vi "DDS_Clock.vi"() -> ()   [LabVIEW 2016] (continued)
 [Hz] CH0"=300199999.99999994}, {"total time[ms]"=89.94999999999703, "f1 [Hz] CH0"=300199999.99999994}, {"total time[ms]"=89.99999999999703, "f1 [Hz] CH0"=300000000.0}, {"total time[ms]"=89.99999999999703, "f1 [Hz] CH0"=300000000.0}, {"total time[ms]"=90.04999999999703, "f1 [Hz] CH0"=300200000.00000006}, {"total time[ms]"=90.04999999999703, "f1 [Hz] CH0"=300200000.00000006}, {"total time[ms]"=90.09999999999702, "f1 [Hz] CH0"=300400000.00000006}, {"total time[ms]"=90.09999999999702, "f1 [Hz] CH0"=300400000.00000006}, {"total time[ms]"=90.14999999999702, "f1 [Hz] CH0"=300600000.0}, {"total time[ms]"=90.14999999999702, "f1 [Hz] CH0"=300600000.0}, {"total time[ms]"=90.19999999999702, "f1 [Hz] CH0"=300800000.00000006}, {"total time[ms]"=90.19999999999702, "f1 [Hz] CH0"=300800000.00000006}, {"total time[ms]"=90.24999999999702, "f1 [Hz] CH0"=301000000.0}, {"total time[ms]"=90.24999999999702, "f1 [Hz] CH0"=301000000.0}, {"total time[ms]"=90.29999999999701, "f1 [Hz] CH0"=301200000.00000006}, {"total time[ms]"=90.29999999999701, "f1 [Hz] CH0"=301200000.00000006}, {"total time[ms]"=90.34999999999701, "f1 [Hz] CH0"=301400000.00000006}, {"total time[ms]"=90.34999999999701, "f1 [Hz] CH0"=301400000.00000006}, {"total time[ms]"=90.39999999999701, "f1 [Hz] CH0"=301600000.00000006}, {"total time[ms]"=90.39999999999701, "f1 [Hz] CH0"=301600000.00000006}, {"total time[ms]"=90.449999999997, "f1 [Hz] CH0"=301800000.0}, {"total time[ms]"=90.449999999997, "f1 [Hz] CH0"=301800000.0}, {"total time[ms]"=90.499999999997, "f1 [Hz] CH0"=302000000.0}, {"total time[ms]"=90.499999999997, "f1 [Hz] CH0"=302000000.0}, {"total time[ms]"=90.549999999997, "f1 [Hz] CH0"=302200000.00000006}, {"total time[ms]"=90.549999999997, "f1 [Hz] CH0"=302200000.00000006}, {"total time[ms]"=90.599999999997, "f1 [Hz] CH0"=302400000.0}, {"total time[ms]"=90.599999999997, "f1 [Hz] CH0"=302400000.0}, {"total time[ms]"=90.649999999997, "f1 [Hz] CH0"=302600000.00000006}, {"total time[ms]"=90.649999999997, "f1 [Hz] CH0"=302600000.00000006}, {"total time[ms]"=90.69999999999699, "f1 [Hz] CH0"=302800000.0}, {"total time[ms]"=90.69999999999699, "f1 [Hz] CH0"=302800000.0}, {"total time[ms]"=90.74999999999699, "f1 [Hz] CH0"=303000000.00000006}, {"total time[ms]"=90.74999999999699, "f1 [Hz] CH0"=303000000.00000006}, {"total time[ms]"=90.79999999999698, "f1 [Hz] CH0"=303200000.00000006}, {"total time[ms]"=90.79999999999698, "f1 [Hz] CH0"=303200000.00000006}, {"total time[ms]"=90.84999999999698, "f1 [Hz] CH0"=303400000.00000006}, {"total time[ms]"=90.84999999999698, "f1 [Hz] CH0"=303400000.00000006}, {"total time[ms]"=90.89999999999698, "f1 [Hz] CH0"=303600000.00000006}, {"total time[ms]"=90.89999999999698, "f1 [Hz] CH0"=303600000.00000006}, {"total time[ms]"=90.94999999999698, "f1 [Hz] CH0"=303800000.0}, {"total time[ms]"=90.94999999999698, "f1 [Hz] CH0"=303800000.0}, {"total time[ms]"=90.99999999999697, "f1 [Hz] CH0"=304000000.0}, {"total time[ms]"=90.99999999999697, "f1 [Hz] CH0"=304000000.0}, {"total time[ms]"=91.04999999999697, "f1 [Hz] CH0"=304200000.00000006}, {"total time[ms]"=91.04999999999697, "f1 [Hz] CH0"=304200000.00000006}, {"total time[ms]"=91.09999999999697, "f1 [Hz] CH0"=304400000.00000006}, {"total time[ms]"=91.09999999999697, "f1 [Hz] CH0"=304400000.00000006}, {"total time[ms]"=91.14999999999696, "f1 [Hz] CH0"=304600000.0}, {"total time[ms]"=91.14999999999696, "f1 [Hz] CH0"=304600000.0}, {"total time[ms]"=91.19999999999696, "f1 [Hz] CH0"=304800000.00000006}, {"total time[ms]"=91.19999999999696, "f1 [Hz] CH0"=304800000.00000006}, {"total time[ms]"=91.24999999999696, "f1 [Hz] CH0"=305000000.0}, {"total time[ms]"=91.24999999999696, "f1 [Hz] CH0"=305000000.0}, {"total time[ms]"=91.29999999999696, "f1 [Hz] CH0"=305200000.00000006}, {"total time[ms]"=91.29999999999696, "f1 [Hz] CH0"=305200000.00000006}, {"total time[ms]"=91.34999999999695, "f1 [Hz] CH0"=305400000.00000006}, {"total time[ms]"=91.34999999999695, "f1 [Hz] CH0"=305400000.00000006}, {"total time[ms]"=91.39999999999695, "f1 [Hz] CH0"=305600000.0}, {"total time[ms]"=91.39999999999695, "f1 [Hz] CH0"=305600000.0}, {"total time[ms]"=91.44999999999695, "f1 [Hz] CH0"=305800000.00000006}, {"total time[ms]"=91.44999999999695, "f1 [Hz] CH0"=305800000.00000006}, {"total time[ms]"=91.49999999999694, "f1 [Hz] CH0"=306000000.0}, {"total time[ms]"=91.49999999999694, "f1 [Hz] CH0"=306000000.0}, {"total time[ms]"=91.54999999999694, "f1 [Hz] CH0"=306200000.00000006}, {"total time[ms]"=91.54999999999694, "f1 [Hz] CH0"=306200000.00000006}, {"total time[ms]"=91.59999999999694, "f1 [Hz] CH0"=306400000.00000006}, {"total time[ms]"=91.59999999999694, "f1 [Hz] CH0"=306400000.00000006}, {"total time[ms]"=91.64999999999694, "f1 [Hz] CH0"=306600000.00000006}, {"total time[ms]"=91.64999999999694, "f1 [Hz] CH0"=306600000.00000006}, {"total time[ms]"=91.69999999999693, "f1 [Hz] CH0"=306800000.0}, {"total time[ms]"=91.69999999999693, "f1 [Hz] CH0"=306800000.0}, {"total time[ms]"=91.74999999999693, "f1 [Hz] CH0"=307000000.0}, {"total time[ms]"=91.74999999999693, "f1 [Hz] CH0"=307000000.0}, {"total time[ms]"=91.79999999999693, "f1 [Hz] CH0"=307200000.00000006}, {"total time[ms]"=91.79999999999693, "f1 [Hz] CH0"=307200000.00000006}, {"total time[ms]"=91.84999999999692, "f1 [Hz] CH0"=307400000.0}, {"total time[ms]"=91.84999999999692, "f1 [Hz] CH0"=307400000.0}, {"total time[ms]"=91.89999999999692, "f1 [Hz] CH0"=307600000.00000006}, {"total time[ms]"=91.89999999999692, "f1 [Hz] CH0"=307600000.00000006}, {"total time[ms]"=91.94999999999692, "f1 [Hz] CH0"=307800000.0}, {"total time[ms]"=91.94999999999692, "f1 [Hz] CH0"=307800000.0}, {"total time[ms]"=91.99999999999692, "f1 [Hz] CH0"=308000000.00000006}, {"total time[ms]"=91.99999999999692, "f1 [Hz] CH0"=308000000.00000006}, {"total time[ms]"=92.04999999999691, "f1 [Hz] CH0"=308200000.00000006}, {"total time[ms]"=92.04999999999691, "f1 [Hz] CH0"=308200000.00000006}, {"total time[ms]"=92.09999999999691, "f1 [Hz] CH0"=308400000.00000006}, {"total time[ms]"=92.09999999999691, "f1 [Hz] CH0"=308400000.00000006}, {"total time[ms]"=92.14999999999691, "f1 [Hz] CH0"=308600000.00000006}, {"total time[ms]"=92.14999999999691, "f1 [Hz] CH0"=308600000.00000006}, {"total time[ms]"=92.1999999999969, "f1 [Hz] CH0"=308800000.0}, {"total time[ms]"=92.1999999999969, "f1 [Hz] CH0"=308800000.0}, {"total time[ms]"=92.2499999999969, "f1 [Hz] CH0"=309000000.0}, {"total time[ms]"=92.2499999999969, "f1 [Hz] CH0"=309000000.0}, {"total time[ms]"=92.2999999999969, "f1 [Hz] CH0"=309200000.00000006}, {"total time[ms]"=92.2999999999969, "f1 [Hz] CH0"=309200000.00000006}, {"total time[ms]"=92.3499999999969, "f1 [Hz] CH0"=309400000.00000006}, {"total time[ms]"=92.3499999999969, "f1 [Hz] CH0"=309400000.00000006}, {"total time[ms]"=92.3999999999969, "f1 [Hz] CH0"=309600000.0}, {"total time[ms]"=92.3999999999969, "f1 [Hz] CH0"=309600000.0}, {"total time[ms]"=92.44999999999689, "f1 [Hz] CH0"=309800000.00000006}, {"total time[ms]"=92.44999999999689, "f1 [Hz] CH0"=309800000.00000006}, {"total time[ms]"=92.49999999999689, "f1 [Hz] CH0"=310000000.0}, {"total time[ms]"=92.49999999999689, "f1 [Hz] CH0"=310000000.0}, {"total time[ms]"=92.54999999999688, "f1 [Hz] CH0"=310200000.00000006}, {"total time[ms]"=92.54999999999688, "f1 [Hz] CH0"=310200000.00000006}, {"total time[ms]"=92.59999999999688, "f1 [Hz] CH0"=310400000.00000006}, {"total time[ms]"=92.59999999999688, "f1 [Hz] CH0"=310400000.00000006}, {"total time[ms]"=92.64999999999688, "f1 [Hz] CH0"=310600000.0}, {"total time[ms]"=92.64999999999688, "f1 [Hz] CH0"=310600000.0}, {"total time[ms]"=92.69999999999688, "f1 [Hz] CH0"=310800000.00000006}, {"total time[ms]"=92.69999999999688, "f1 [Hz] CH0"=310800000.00000006}, {"total time[ms]"=92.74999999999687, "f1 [Hz] CH0"=311000000.0}, {"total time[ms]"=92.74999999999687, "f1 [Hz] CH0"=311000000.0}, {"total time[ms]"=92.79999999999687, "f1 [Hz] CH0"=311200000.00000006}, {"total time[ms]"=92.79999999999687, "f1 [Hz] CH0"=311200000.00000006}, {"total time[ms]"=92.84999999999687, "f1 [Hz] CH0"=311400000.00000006}, {"total time[ms]"=92.84999999999687, "f1 [Hz] CH0"=311400000.00000006}, {"total time[ms]"=92.89999999999687, "f1 [Hz] CH0"=311600000.00000006}, {"total time[ms]"=92.89999999999687, "f1 [Hz] CH0"=311600000.00000006}, {"total time[ms]"=92.94999999999686, "f1 [Hz] CH0"=311800000.0}, {"total time[ms]"=92.94999999999686, "f1 [Hz] CH0"=311800000.0}, {"total time[ms]"=92.99999999999686, "f1 [Hz] CH0"=312000000.0}, {"total time[ms]"=92.99999999999686, "f1 [Hz] CH0"=312000000.0}, {"total time[ms]"=93.04999999999686, "f1 [Hz] CH0"=312200000.00000006}, {"total time[ms]"=93.04999999999686, "f1 [Hz] CH0"=312200000.00000006}, {"total time[ms]"=93.09999999999685, "f1 [Hz] CH0"=312400000.0}, {"total time[ms]"=93.09999999999685, "f1 [Hz] CH0"=312400000.0}, {"total time[ms]"=93.14999999999685, "f1 [Hz] CH0"=312600000.00000006}, {"total time[ms]"=93.14999999999685, "f1 [Hz] CH0"=312600000.00000006}, {"total time[ms]"=93.19999999999685, "f1 [Hz] CH0"=312800000.0}, {"total time[ms]"=93.19999999999685, "f1 [Hz] CH0"=312800000.0}, {"total time[ms]"=93.24999999999685, "f1 [Hz] CH0"=313000000.00000006}, {"total time[ms]"=93.24999999999685, "f1 [Hz] CH0"=313000000.00000006}, {"total time[ms]"=93.29999999999684, "f1 [Hz] CH0"=313200000.00000006}, {"total time[ms]"=93.29999999999684, "f1 [Hz] CH0"=313200000.00000006}, {"total time[ms]"=93.34999999999684, "f1 [Hz] CH0"=313400000.00000006}, {"total time[ms]"=93.34999999999684, "f1 [Hz] CH0"=313400000.00000006}, {"total time[ms]"=93.39999999999684, "f1 [Hz] CH0"=313600000.00000006}, {"total time[ms]"=93.39999999999684, "f1 [Hz] CH0"=313600000.00000006}, {"total time[ms]"=93.44999999999683, "f1 [Hz] CH0"=313800000.0}, {"total time[ms]"=93.44999999999683, "f1 [Hz] CH0"=313800000.0}, {"total time[ms]"=93.49999999999683, "f1 [Hz] CH0"=314000000.0}, {"total time[ms]"=93.49999999999683, "f1 [Hz] CH0"=314000000.0}, {"total time[ms]"=93.54999999999683, "f1 [Hz] CH0"=314200000.00000006}, {"total time[ms]"=93.54999999999683, "f1 [Hz] CH0"=314200000.00000006}, {"total time[ms]"=93.59999999999683, "f1 [Hz] CH0"=314400000.00000006}, {"total time[ms]"=93.59999999999683, "f1 [Hz] CH0"=314400000.00000006}, {"total time[ms]"=93.64999999999682, "f1 [Hz] CH0"=314600000.0}, {"total time[ms]"=93.64999999999682, "f1 [Hz] CH0"=314600000.0}, {"total time[ms]"=93.69999999999682, "f1 [Hz] CH0"=314800000.00000006}, {"total time[ms]"=93.69999999999682, "f1 [Hz] CH0"=314800000.00000006}, {"total time[ms]"=93.74999999999682, "f1 [Hz] CH0"=315000000.0}, {"total time[ms]"=93.74999999999682, "f1 [Hz] CH0"=315000000.0}, {"total time[ms]"=93.79999999999681, "f1 [Hz] CH0"=315200000.00000006}, {"total time[ms]"=93.79999999999681, "f1 [Hz] CH0"=315200000.00000006}, {"total time[ms]"=93.84999999999681, "f1 [Hz] CH0"=315400000.00000006}, {"total time[ms]"=93.84999999999681, "f1 [Hz] CH0"=315400000.00000006}, {"total time[ms]"=93.89999999999681, "f1 [Hz] CH0"=315600000.0}, {"total time[ms]"=93.89999999999681, "f1 [Hz] CH0"=315600000.0}, {"total time[ms]"=93.9499999999968, "f1 [Hz] CH0"=315800000.00000006}, {"total time[ms]"=93.9499999999968, "f1 [Hz] CH0"=315800000.00000006}, {"total time[ms]"=93.9999999999968, "f1 [Hz] CH0"=316000000.0}, {"total time[ms]"=93.9999999999968, "f1 [Hz] CH0"=316000000.0}, {"total time[ms]"=94.0499999999968, "f1 [Hz] CH0"=316200000.00000006}, {"total time[ms]"=94.0499999999968, "f1 [Hz] CH0"=316200000.00000006}, {"total time[ms]"=94.0999999999968, "f1 [Hz] CH0"=316400000.00000006}, {"total time[ms]"=94.0999999999968, "f1 [Hz] CH0"=316400000.00000006}, {"total time[ms]"=94.1499999999968, "f1 [Hz] CH0"=316600000.00000006}, {"total time[ms]"=94.1499999999968, "f1 [Hz] CH0"=316600000.00000006}, {"total time[ms]"=94.19999999999679, "f1 [Hz] CH0"=316800000.0}, {"total time[ms]"=94.19999999999679, "f1 [Hz] CH0"=316800000.0}, {"total time[ms]"=94.24999999999679, "f1 [Hz] CH0"=317000000.0}, {"total time[ms]"=94.24999999999679, "f1 [Hz] CH0"=317000000.0}, {"total time[ms]"=94.29999999999679, "f1 [Hz] CH0"=317200000.00000006}, {"total time[ms]"=94.29999999999679, "f1 [Hz] CH0"=317200000.00000006}, {"total time[ms]"=94.34999999999678, "f1 [Hz] CH0"=317400000.0}, {"total time[ms]"=94.34999999999678, "f1 [Hz] CH0"=317400000.0}, {"total time[ms]"=94.39999999999678, "f1 [Hz] CH0"=317600000.00000006}, {"total time[ms]"=94.39999999999678, "f1 [Hz] CH0"=317600000.00000006}, {"total time[ms]"=94.44999999999678, "f1 [Hz] CH0"=317800000.0}, {"total time[ms]"=94.44999999999678, "f1 [Hz] CH0"=317800000.0}, {"total time[ms]"=94.49999999999677, "f1 [Hz] CH0"=318000000.00000006}, {"total time[ms]"=94.49999999999677, "f1 [Hz] CH0"=318000000.00000006}, {"total time[ms]"=94.54999999999677, "f1 [Hz] CH0"=318200000.00000006}, {"total time[ms]"=94.54999999999677, "f1 [Hz] CH0"=318200000.00000006}, {"total time[ms]"=94.59999999999677, "f1 [Hz] CH0"=318400000.00000006}, {"total time[ms]"=94.59999999999677, "f1 [Hz] CH0"=318400000.00000006}, {"total time[ms]"=94.64999999999677, "f1 [Hz] CH0"=318600000.00000006}, {"total time[ms]"=94.64999999999677, "f1 [Hz] CH0"=318600000.00000006}, {"total time[ms]"=94.69999999999676, "f1 [Hz] CH0"=318800000.0}, {"total time[ms]"=94.69999999999676, "f1 [Hz] CH0"=318800000.0}, {"total time[ms]"=94.74999999999676, "f1 [Hz] CH0"=319000000.0}, {"total time[ms]"=94.74999999999676, "f1 [Hz] CH0"=319000000.0}, {"total time[ms]"=94.79999999999676, "f1 [Hz] CH0"=319200000.0000001}, {"total time[ms]"=94.79999999999676, "f1 [Hz] CH0"=319200000.0000001}, {"total time[ms]"=94.84999999999675, "f1 [Hz] CH0"=319400000.00000006}, {"total time[ms]"=94.84999999999675, "f1 [Hz] CH0"=319400000.00000006}, {"total time[ms]"=94.89999999999675, "f1 [Hz] CH0"=319600000.0}, {"total time[ms]"=94.89999999999675, "f1 [Hz] CH0"=319600000.0}, {"total time[ms]"=94.94999999999675, "f1 [Hz] CH0"=319800000.00000006}, {"total time[ms]"=94.94999999999675, "f1 [Hz] CH0"=319800000.00000006}, {"total time[ms]"=94.99999999999675, "f1 [Hz] CH0"=320000000.0}, {"total time[ms]"=94.99999999999675, "f1 [Hz] CH0"=320000000.0}, {"total time[ms]"=95.04999999999674, "f1 [Hz] CH0"=319800000.0}, {"total time[ms]"=95.04999999999674, "f1 [Hz] CH0"=319800000.0}, {"total time[ms]"=95.09999999999674, "f1 [Hz] CH0"=319599999.99999994}, {"total time[ms]"=95.09999999999674, "f1 [Hz] CH0"=319599999.99999994}, {"total time[ms]"=95.14999999999674, "f1 [Hz] CH0"=319400000.0}, {"total time[ms]"=95.14999999999674, "f1 [Hz] CH0"=319400000.0}, {"total time[ms]"=95.19999999999673, "f1 [Hz] CH0"=319199999.99999994}, {"total time[ms]"=95.19999999999673, "f1 [Hz] CH0"=319199999.99999994}, {"total time[ms]"=95.24999999999673, "f1 [Hz] CH0"=319000000.0}, {"total time[ms]"=95.24999999999673, "f1 [Hz] CH0"=319000000.0}, {"total time[ms]"=95.29999999999673, "f1 [Hz] CH0"=318799999.99999994}, {"total time[ms]"=95.29999999999673, "f1 [Hz] CH0"=318799999.99999994}, {"total time[ms]"=95.34999999999673, "f1 [Hz] CH0"=318599999.99999994}, {"total time[ms]"=95.34999999999673, "f1 [Hz] CH0"=318599999.99999994}, {"total time[ms]"=95.39999999999672, "f1 [Hz] CH0"=318399999.99999994}, {"total time[ms]"=95.39999999999672, "f1 [Hz] CH0"=318399999.99999994}, {"total time[ms]"=95.44999999999672, "f1 [Hz] CH0"=318200000.0}, {"total time[ms]"=95.44999999999672, "f1 [Hz] CH0"=318200000.0}, {"total time[ms]"=95.49999999999672, "f1 [Hz] CH0"=318000000.0}, {"total time[ms]"=95.49999999999672, "f1 [Hz] CH0"=318000000.0}, {"total time[ms]"=95.54999999999671, "f1 [Hz] CH0"=317799999.99999994}, {"total time[ms]"=95.54999999999671, "f1 [Hz] CH0"=317799999.99999994}, {"total time[ms]"=95.59999999999671, "f1 [Hz] CH0"=317600000.0}, {"total time[ms]"=95.59999999999671, "f1 [Hz] CH0"=317600000.0}, {"total time[ms]"=95.64999999999671, "f1 [Hz] CH0"=317399999.99999994}, {"total time[ms]"=95.64999999999671, "f1 [Hz] CH0"=317399999.99999994}, {"total time[ms]"=95.6999999999967, "f1 [Hz] CH0"=317200000.0}, {"total time[ms]"=95.6999999999967, "f1 [Hz] CH0"=317200000.0}, {"total time[ms]"=95.7499999999967, "f1 [Hz] CH0"=316999999.99999994}, {"total time[ms]"=95.7499999999967, "f1 [Hz] CH0"=316999999.99999994}, {"total time[ms]"=95.7999999999967, "f1 [Hz] CH0"=316799999.99999994}, {"total time[ms]"=95.7999999999967, "f1 [Hz] CH0"=316799999.99999994}, {"total time[ms]"=95.8499999999967, "f1 [Hz] CH0"=316599999.99999994}, {"total time[ms]"=95.8499999999967, "f1 [Hz] CH0"=316599999.99999994}, {"total time[ms]"=95.8999999999967, "f1 [Hz] CH0"=316399999.99999994}, {"total time[ms]"=95.8999999999967, "f1 [Hz] CH0"=316399999.99999994}, {"total time[ms]"=95.94999999999669, "f1 [Hz] CH0"=316200000.0}, {"total time[ms]"=95.94999999999669, "f1 [Hz] CH0"=316200000.0}, {"total time[ms]"=95.99999999999669, "f1 [Hz] CH0"=315999999.99999994}, {"total time[ms]"=95.99999999999669, "f1 [Hz] CH0"=315999999.99999994}, {"total time[ms]"=96.04999999999669, "f1 [Hz] CH0"=315799999.99999994}, {"total time[ms]"=96.04999999999669, "f1 [Hz] CH0"=315799999.99999994}, {"total time[ms]"=96.09999999999668, "f1 [Hz] CH0"=315599999.99999994}, {"total time[ms]"=96.09999999999668, "f1 [Hz] CH0"=315599999.99999994}, {"total time[ms]"=96.14999999999668, "f1 [Hz] CH0"=315399999.99999994}, {"total time[ms]"=96.14999999999668, "f1 [Hz] CH0"=315399999.99999994}, {"total time[ms]"=96.19999999999668, "f1 [Hz] CH0"=315199999.99999994}, {"total time[ms]"=96.19999999999668, "f1 [Hz] CH0"=315199999.99999994}, {"total time[ms]"=96.24999999999667, "f1 [Hz] CH0"=315000000.0}, {"total time[ms]"=96.24999999999667, "f1 [Hz] CH0"=315000000.0}, {"total time[ms]"=96.29999999999667, "f1 [Hz] CH0"=314799999.9999999}, {"total time[ms]"=96.29999999999667, "f1 [Hz] CH0"=314799999.9999999}, {"total time[ms]"=96.34999999999667, "f1 [Hz] CH0"=314599999.99999994}, {"total time[ms]"=96.34999999999667, "f1 [Hz] CH0"=314599999.99999994}, {"total time[ms]"=96.39999999999667, "f1 [Hz] CH0"=314400000.0}, {"total time[ms]"=96.39999999999667, "f1 [Hz] CH0"=314400000.0}, {"total time[ms]"=96.44999999999666, "f1 [Hz] CH0"=314199999.99999994}, {"total time[ms]"=96.44999999999666, "f1 [Hz] CH0"=314199999.99999994}, {"total time[ms]"=96.49999999999666, "f1 [Hz] CH0"=314000000.0}, {"total time[ms]"=96.49999999999666, "f1 [Hz] CH0"=314000000.0}, {"total time[ms]"=96.54999999999666, "f1 [Hz] CH0"=313799999.99999994}, {"total time[ms]"=96.54999999999666, "f1 [Hz] CH0"=313799999.99999994}, {"total time[ms]"=96.59999999999665, "f1 [Hz] CH0"=313599999.99999994}, {"total time[ms]"=96.59999999999665, "f1 [Hz] CH0"=313599999.99999994}, {"total time[ms]"=96.64999999999665, "f1 [Hz] CH0"=313399999.99999994}, {"total time[ms]"=96.64999999999665, "f1 [Hz] CH0"=313399999.99999994}, {"total time[ms]"=96.69999999999665, "f1 [Hz] CH0"=313199999.99999994}, {"total time[ms]"=96.69999999999665, "f1 [Hz] CH0"=313199999.99999994}, {"total time[ms]"=96.74999999999665, "f1 [Hz] CH0"=313000000.0}, {"total time[ms]"=96.74999999999665, "f1 [Hz] CH0"=313000000.0}, {"total time[ms]"=96.79999999999664, "f1 [Hz] CH0"=312799999.99999994}, {"total time[ms]"=96.79999999999664, "f1 [Hz] CH0"=312799999.99999994}, {"total time[ms]"=96.84999999999664, "f1 [Hz] CH0"=312599999.9999999}, {"total time[ms]"=96.84999999999664, "f1 [Hz] CH0"=312599999.9999999}, {"total time[ms]"=96.89999999999664, "f1 [Hz] CH0"=312399999.99999994}, {"total time[ms]"=96.89999999999664, "f1 [Hz] CH0"=312399999.99999994}, {"total time[ms]"=96.94999999999663, "f1 [Hz] CH0"=312200000.0}, {"total time[ms]"=96.94999999999663, "f1 [Hz] CH0"=312200000.0}, {"total time[ms]"=96.99999999999663, "f1 [Hz] CH0"=311999999.99999994}, {"total time[ms]"=96.99999999999663, "f1 [Hz] CH0"=311999999.99999994}, {"total time[ms]"=97.04999999999663, "f1 [Hz] CH0"=311799999.99999994}, {"total time[ms]"=97.04999999999663, "f1 [Hz] CH0"=311799999.99999994}, {"total time[ms]"=97.09999999999663, "f1 [Hz] CH0"=311599999.99999994}, {"total time[ms]"=97.09999999999663, "f1 [Hz] CH0"=311599999.99999994}, {"total time[ms]"=97.14999999999662, "f1 [Hz] CH0"=311399999.99999994}, {"total time[ms]"=97.14999999999662, "f1 [Hz] CH0"=311399999.99999994}, {"total time[ms]"=97.19999999999662, "f1 [Hz] CH0"=311200000.0}, {"total time[ms]"=97.19999999999662, "f1 [Hz] CH0"=311200000.0}, {"total time[ms]"=97.24999999999662, "f1 [Hz] CH0"=310999999.99999994}, {"total time[ms]"=97.24999999999662, "f1 [Hz] CH0"=310999999.99999994}, {"total time[ms]"=97.29999999999661, "f1 [Hz] CH0"=310799999.99999994}, {"total time[ms]"=97.29999999999661, "f1 [Hz] CH0"=310799999.99999994}, {"total time[ms]"=97.34999999999661, "f1 [Hz] CH0"=310599999.99999994}, {"total time[ms]"=97.34999999999661, "f1 [Hz] CH0"=310599999.99999994}, {"total time[ms]"=97.39999999999661, "f1 [Hz] CH0"=310399999.99999994}, {"total time[ms]"=97.39999999999661, "f1 [Hz] CH0"=310399999.99999994}, {"total time[ms]"=97.4499999999966, "f1 [Hz] CH0"=310199999.99999994}, {"total time[ms]"=97.4499999999966, "f1 [Hz] CH0"=310199999.99999994}, {"total time[ms]"=97.4999999999966, "f1 [Hz] CH0"=310000000.0}, {"total time[ms]"=97.4999999999966, "f1 [Hz] CH0"=310000000.0}, {"total time[ms]"=97.5499999999966, "f1 [Hz] CH0"=309799999.9999999}, {"total time[ms]"=97.5499999999966, "f1 [Hz] CH0"=309799999.9999999}, {"total time[ms]"=97.5999999999966, "f1 [Hz] CH0"=309599999.99999994}, {"total time[ms]"=97.5999999999966, "f1 [Hz] CH0"=309599999.99999994}, {"total time[ms]"=97.6499999999966, "f1 [Hz] CH0"=309400000.0}, {"total time[ms]"=97.6499999999966, "f1 [Hz] CH0"=309400000.0}, {"total time[ms]"=97.69999999999659, "f1 [Hz] CH0"=309199999.99999994}, {"total time[ms]"=97.69999999999659, "f1 [Hz] CH0"=309199999.99999994}, {"total time[ms]"=97.74999999999659, "f1 [Hz] CH0"=309000000.0}, {"total time[ms]"=97.74999999999659, "f1 [Hz] CH0"=309000000.0}, {"total time[ms]"=97.79999999999659, "f1 [Hz] CH0"=308799999.99999994}, {"total time[ms]"=97.79999999999659, "f1 [Hz] CH0"=308799999.99999994}, {"total time[ms]"=97.84999999999658, "f1 [Hz] CH0"=308599999.99999994}, {"total time[ms]"=97.84999999999658, "f1 [Hz] CH0"=308599999.99999994}, {"total time[ms]"=97.89999999999658, "f1 [Hz] CH0"=308399999.99999994}, {"total time[ms]"=97.89999999999658, "f1 [Hz] CH0"=308399999.99999994}, {"total time[ms]"=97.94999999999658, "f1 [Hz] CH0"=308199999.99999994}, {"total time[ms]"=97.94999999999658, "f1 [Hz] CH0"=308199999.99999994}, {"total time[ms]"=97.99999999999658, "f1 [Hz] CH0"=308000000.0}, {"total time[ms]"=97.99999999999658, "f1 [Hz] CH0"=308000000.0}, {"total time[ms]"=98.04999999999657, "f1 [Hz] CH0"=307799999.99999994}, {"total time[ms]"=98.04999999999657, "f1 [Hz] CH0"=307799999.99999994}, {"total time[ms]"=98.09999999999657, "f1 [Hz] CH0"=307599999.9999999}, {"total time[ms]"=98.09999999999657, "f1 [Hz] CH0"=307599999.9999999}, {"total time[ms]"=98.14999999999657, "f1 [Hz] CH0"=307399999.99999994}, {"total time[ms]"=98.14999999999657, "f1 [Hz] CH0"=307399999.99999994}, {"total time[ms]"=98.19999999999656, "f1 [Hz] CH0"=307200000.0}, {"total time[ms]"=98.19999999999656, "f1 [Hz] CH0"=307200000.0}, {"total time[ms]"=98.24999999999656, "f1 [Hz] CH0"=306999999.99999994}, {"total time[ms]"=98.24999999999656, "f1 [Hz] CH0"=306999999.99999994}, {"total time[ms]"=98.29999999999656, "f1 [Hz] CH0"=306799999.99999994}, {"total time[ms]"=98.29999999999656, "f1 [Hz] CH0"=306799999.99999994}, {"total time[ms]"=98.34999999999656, "f1 [Hz] CH0"=306599999.99999994}, {"total time[ms]"=98.34999999999656, "f1 [Hz] CH0"=306599999.99999994}, {"total time[ms]"=98.39999999999655, "f1 [Hz] CH0"=306399999.99999994}, {"total time[ms]"=98.39999999999655, "f1 [Hz] CH0"=306399999.99999994}, {"total time[ms]"=98.44999999999655, "f1 [Hz] CH0"=306200000.0}, {"total time[ms]"=98.44999999999655, "f1 [Hz] CH0"=306200000.0}, {"total time[ms]"=98.49999999999655, "f1 [Hz] CH0"=305999999.99999994}, {"total time[ms]"=98.49999999999655, "f1 [Hz] CH0"=305999999.99999994}, {"total time[ms]"=98.54999999999654, "f1 [Hz] CH0"=305799999.99999994}, {"total time[ms]"=98.54999999999654, "f1 [Hz] CH0"=305799999.99999994}, {"total time[ms]"=98.59999999999654, "f1 [Hz] CH0"=305599999.99999994}, {"total time[ms]"=98.59999999999654, "f1 [Hz] CH0"=305599999.99999994}, {"total time[ms]"=98.64999999999654, "f1 [Hz] CH0"=305399999.99999994}, {"total time[ms]"=98.64999999999654, "f1 [Hz] CH0"=305399999.99999994}, {"total time[ms]"=98.69999999999654, "f1 [Hz] CH0"=305199999.99999994}, {"total time[ms]"=98.69999999999654, "f1 [Hz] CH0"=305199999.99999994}, {"total time[ms]"=98.74999999999653, "f1 [Hz] CH0"=305000000.0}, {"total time[ms]"=98.74999999999653, "f1 [Hz] CH0"=305000000.0}, {"total time[ms]"=98.79999999999653, "f1 [Hz] CH0"=304799999.9999999}, {"total time[ms]"=98.79999999999653, "f1 [Hz] CH0"=304799999.9999999}, {"total time[ms]"=98.84999999999653, "f1 [Hz] CH0"=304599999.99999994}, {"total time[ms]"=98.84999999999653, "f1 [Hz] CH0"=304599999.99999994}, {"total time[ms]"=98.89999999999652, "f1 [Hz] CH0"=304400000.0}, {"total time[ms]"=98.89999999999652, "f1 [Hz] CH0"=304400000.0}, {"total time[ms]"=98.94999999999652, "f1 [Hz] CH0"=304199999.99999994}, {"total time[ms]"=98.94999999999652, "f1 [Hz] CH0"=304199999.99999994}, {"total time[ms]"=98.99999999999652, "f1 [Hz] CH0"=304000000.0}, {"total time[ms]"=98.99999999999652, "f1 [Hz] CH0"=304000000.0}, {"total time[ms]"=99.04999999999652, "f1 [Hz] CH0"=303799999.99999994}, {"total time[ms]"=99.04999999999652, "f1 [Hz] CH0"=303799999.99999994}, {"total time[ms]"=99.09999999999651, "f1 [Hz] CH0"=303599999.99999994}, {"total time[ms]"=99.09999999999651, "f1 [Hz] CH0"=303599999.99999994}, {"total time[ms]"=99.14999999999651, "f1 [Hz] CH0"=303399999.99999994}, {"total time[ms]"=99.14999999999651, "f1 [Hz] CH0"=303399999.99999994}, {"total time[ms]"=99.1999999999965, "f1 [Hz] CH0"=303199999.99999994}, {"total time[ms]"=99.1999999999965, "f1 [Hz] CH0"=303199999.99999994}, {"total time[ms]"=99.2499999999965, "f1 [Hz] CH0"=303000000.0}, {"total time[ms]"=99.2499999999965, "f1 [Hz] CH0"=303000000.0}, {"total time[ms]"=99.2999999999965, "f1 [Hz] CH0"=302799999.99999994}, {"total time[ms]"=99.2999999999965, "f1 [Hz] CH0"=302799999.99999994}, {"total time[ms]"=99.3499999999965, "f1 [Hz] CH0"=302599999.9999999}, {"total time[ms]"=99.3499999999965, "f1 [Hz] CH0"=302599999.9999999}, {"total time[ms]"=99.3999999999965, "f1 [Hz] CH0"=302399999.99999994}, {"total time[ms]"=99.3999999999965, "f1 [Hz] CH0"=302399999.99999994}, {"total time[ms]"=99.44999999999649, "f1 [Hz] CH0"=302200000.0}, {"total time[ms]"=99.44999999999649, "f1 [Hz] CH0"=302200000.0}, {"total time[ms]"=99.49999999999649, "f1 [Hz] CH0"=301999999.99999994}, {"total time[ms]"=99.49999999999649, "f1 [Hz] CH0"=301999999.99999994}, {"total time[ms]"=99.54999999999649, "f1 [Hz] CH0"=301799999.99999994}, {"total time[ms]"=99.54999999999649, "f1 [Hz] CH0"=301799999.99999994}, {"total time[ms]"=99.59999999999648, "f1 [Hz] CH0"=301599999.99999994}, {"total time[ms]"=99.59999999999648, "f1 [Hz] CH0"=301599999.99999994}, {"total time[ms]"=99.64999999999648, "f1 [Hz] CH0"=301399999.99999994}, {"total time[ms]"=99.64999999999648, "f1 [Hz] CH0"=301399999.99999994}, {"total time[ms]"=99.69999999999648, "f1 [Hz] CH0"=301200000.0}, {"total time[ms]"=99.69999999999648, "f1 [Hz] CH0"=301200000.0}, {"total time[ms]"=99.74999999999648, "f1 [Hz] CH0"=300999999.99999994}, {"total time[ms]"=99.74999999999648, "f1 [Hz] CH0"=300999999.99999994}, {"total time[ms]"=99.79999999999647, "f1 [Hz] CH0"=300799999.99999994}, {"total time[ms]"=99.79999999999647, "f1 [Hz] CH0"=300799999.99999994}, {"total time[ms]"=99.84999999999647, "f1 [Hz] CH0"=300599999.99999994}, {"total time[ms]"=99.84999999999647, "f1 [Hz] CH0"=300599999.99999994}, {"total time[ms]"=99.89999999999647, "f1 [Hz] CH0"=300399999.99999994}, {"total time[ms]"=99.89999999999647, "f1 [Hz] CH0"=300399999.99999994}, {"total time[ms]"=99.94999999999646, "f1 [Hz] CH0"=300199999.99999994}, {"total time[ms]"=99.94999999999646, "f1 [Hz] CH0"=300199999.99999994}, {"total time[ms]"=99.99999999999646, "f1 [Hz] CH0"=300000000.0}, {"total time[ms]"=99.99999999999646, "f1 [Hz] CH0"=300000000.0}, {"total time[ms]"=100.04999999999646, "f1 [Hz] CH0"=300200000.0000001}]}, ...(2 in all)]
  in  "Store data":enum32{"Save settings", "Don't save settings"}(tab)=enum."Don't save settings"
  in  "XML File Path WRITE":path=path "U:/Dokumente/Bachelorarbeit/Labview/FlexDDS-NG/conf/settings_s_curve_up_down.xml"
  in  "Select curve form":enum32{"Triangular", "Sinusodial"}(ring)
  in  "Single Frequency (MHz)":dbl=310.0 format="%#_13g"
  in  "Channel - Constant":T7(ring)
  in  "Ramping Parameters":T8={"Number of steps"=2000, "Total Time (ms)"=100.0, "Start frequency (MHz)"=300.0, "End frequency (MHz)"=320.0, "Cycle Time (ms)"=10.0} {"Cycle Time (ms)" format="%#_13g"}
  # "Channel - Ramp"
  # "STEP"
  # "time [ms]"
  # "time tolerance [us]"
  # "CH0 [false=wait, keep phase&amplitude]"
  # "rel. amplitude CH0"
  # "phase [°] CH0"
  # "f0 [Hz] CH0"
  # "f1 [Hz] CH0"
  # "CH1 [false=wait, keep phase&amplitude]"
  # "rel. amplitude CH1"
  # "phase [°] CH1"
  # "f0 [Hz] CH1"
  # "f1 [Hz] CH1"
types:
  T1 = enum16{"no_trigger", "BNC_IN_A_RISING", "BNC_IN_A_FALLING", "BNC_IN_B_RISING", "BNC_IN_B_FALLING", "BNC_IN_C_RISING", "BNC_IN_C_FALLING"}
  T2 = cluster{"RAM enable (F)":bool, "Manual OSK external control (F)":bool, "Inverse sinc filter enable (T)":bool, "DDS sine (/cosine) output (F)":bool, "Load LRR at I/O update (F)":bool, "Autoclear digital ramp accumulator (F)":bool, "Autoclear phase accumulator (F)":bool, "Clear digital ramp accumulator (F)":bool, "Clear phase accumulator (F)":bool, "Load ARR at I/O update (F)":bool, "OSK enable (F)":bool, "Select Auto OSK (F)":bool}
  T3 = cluster{"Enable ASF from STP (F)":bool, "Digital ramp enable (F)":bool, "Digital ramp no-dwell high (F)":bool, "Digital ramp no-dwell low (F)":bool, "Matched latency enable (T)":bool, "Parallel data port enable (F)":bool}
  T4 = enum32{"Read from file", "Manual Input", "Generate data with function"}
  T5 = cluster{"STEP":i32, "time[ms]":dbl, "time tolerance[us]":dbl, "CH0":bool, "rel. amplitude CH0":dbl, "phase [°] CH0":dbl, "f0 [Hz] CH0":dbl, "f1 [Hz] CH0":dbl, "CH1":bool, "rel. amplitude CH1":dbl, "phase [°] CH1":dbl, "f0 [Hz] CH1":dbl, "f1 [Hz] CH1":dbl}[]
  T6 = cluster{cluster{"total time[ms]":dbl, "f1 [Hz] CH0":dbl}[]}[]
  T7 = enum16{"Channel CH1 constant", "Channel CH0 constant"}
  T8 = cluster{"Number of steps":i32, "Total Time (ms)":dbl, "Start frequency (MHz)":dbl, "End frequency (MHz)":dbl, "Cycle Time (ms)":dbl}
  T9 = cluster{i32, dbl, "time tolerance":dbl, bool, dbl, dbl, "constant frequency":dbl, "constant frequency":dbl, bool, dbl, dbl, "constant frequency":dbl, "constant frequency":dbl}[]
  T10 = cluster{i32, dbl, "time tolerance":dbl, bool, "Amplitude (Ch 0) ":dbl, "Phase (Ch 0)":dbl, dbl, dbl, bool, "Amplitude (Ch 1) ":dbl, "Phase (Ch 1)":dbl, dbl, dbl}
  T11 = cluster{i32, dbl, "time tolerance":dbl, bool, "Amplitude (Ch 0) ":dbl, "Phase (Ch 0)":dbl, dbl, dbl, bool, "Amplitude (Ch 1) ":dbl, "Phase (Ch 1)":dbl, dbl, dbl}[]
  T12 = cluster{i32, dbl, "time tolerance":dbl, bool, "Amplitude (Ch 0) ":dbl, "Phase (Ch 0)":dbl, "constant frequency":dbl, "constant frequency":dbl, bool, "Amplitude (Ch 1) ":dbl, "Phase (Ch 1)":dbl, "constant frequency":dbl, "constant frequency":dbl}[]
  T13 = cluster{"total time[ms]":dbl, "f1 [Hz] CH1":dbl}[]
  T14 = cluster{"total time[ms]":dbl, "f1 [Hz] CH0":dbl}[]
  T15 = cluster{"STEP":i32, "time[ms]":dbl, "time tolerance[us]":dbl, "CH0":bool, "rel. amplitude CH0":dbl, "phase [°] CH0":dbl, "f0 [Hz] CH0":dbl, "f1 [Hz] CH0":dbl, "CH1":bool, "rel. amplitude CH1":dbl, "phase [°] CH1":dbl, "f0 [Hz] CH1":dbl, "f1 [Hz] CH1":dbl}
  T16 = cluster{"Array":cluster{"total time[ms]":dbl, "f1 [Hz] CH0":dbl}[]}
  T17 = cluster{"Array":cluster{"total time[ms]":dbl, "f1 [Hz] CH1":dbl}[]}
  T18 = cluster{"Array":cluster{"total time[ms]":dbl, "f1 [Hz] CH1":dbl}[]}[]
  T19 = enum32{"Channel 0", "Channel 1", "Both channels"}
  T20 = enum32{"O_RAMP_SWP_OVR", "RAM_SWP_OVR", "O_DROVER", "DROVER", "O_SPI_FIFO_EV1", "SPI_FIFO_EV1", "O_SPI_FIFO_EV0", "SPI_FIFO_EV0", "O_SPI_FIFO_FLUSHED", "SPI_FIFO_FLUSHED", "BNC_IN_B_LEVEL", "BNC_IN_B_FALLING", "BNC_IN_B_RISING", "BNC_IN_A_LEVEL", "BNC_IN_A_FALLING", "BNC_IN_A_RISING", "ALL_SPI_FIFOS_FLUSHED", "NONE"}
diagram:
  n1 = stacked-sequence {
    tunnel: [w35] -> w20
    frame #0 {
      n2 = Unbundle("Ramping Parameters") -> ("Number of steps"=w31:i32, "Total Time (ms)"=w33:dbl, "Start frequency (MHz)"=w23:dbl, "End frequency (MHz)"=w27:dbl, "Cycle Time (ms)"=w29:dbl)
      n3 = Multiply(x=w23, y=1000000.0) -> (x*y=w24:dbl)
      n4 = Multiply(x=w27, y=1000000.0) -> (x*y=w26:dbl)
      n5 = Increment(x=w31) -> (x+1=w30:i32)
      n6 = for {
        N: w30 -> [w44]
        tunnel: w33 -> [w60]
        tunnel: w24 -> [w68]
        tunnel: w26 -> [w69]
        shift-right: [w45] -> w35
        shift-left: T9 [] -> [w46]
        tunnel: w29 -> [w41]
        i -> [w63]
        w73 = 0.01  # time tolerance
        n7 = Decrement(x=w44) -> (x-1=w70:i32)
        n8 = Increment(x=w63) -> (x+1=w62:i32)
        n9 = Build Array(w63, w62) -> (w61:i32[])
        n10 = Divide(x=w60, y=w70) -> (x/y=w43:dbl)
        n11 = Multiply(x=w43, y=w61) -> (x*y=w67:dbl[])
        n12 = case shown="\"Sinusodial\"" "Select curve form" {
          tunnel: w69 -> [w102 w107]
          tunnel: w68 -> [w101 w106]
          tunnel: w67 -> [w94 w113]
          tunnel: w41 -> [w98 w114]
          tunnel: [w86 w103] -> w59
          frame "Sinusodial" {
            n13 = Multiply(x=3.141592653589793, y=2.0) -> (x*y=w96:dbl)
            n14 = Reciprocal(x=w98) -> (1/x=w97:dbl)
            n15 = Multiply(x=w96, y=w97) -> (x*y=w95:dbl)
            n16 = Multiply(x=w94, y=w95) -> (x*y=w93:dbl[])
            n17 = Sine(x=w93) -> (sin(x)=w92:dbl[])
            n18 = Subtract(x=w102, y=w101) -> (x-y=w91:dbl)
            n19 = Multiply(x=w91, y=w92) -> (x*y=w90:dbl[])
            n20 = Add(x=w101, y=w102) -> (x+y=w89:dbl)
            n21 = Subtract(x=w89, y=w90) -> (x-y=w88:dbl[])
            n22 = Divide(x=w88, y=2.0) -> (x/y=w86:dbl[])
          }
          frame "Triangular", Default {
            n23 = Reciprocal(x=w114) -> (1/x=w115:dbl)
            n24 = Multiply(x=w115, y=w113) -> (x*y=w112:dbl[])
            n25 = Round To Nearest(number=w112) -> (nearest integer value=w116:dbl[])
            n26 = Subtract(x=w106, y=w107) -> (x-y=w110:dbl)
            n27 = Subtract(x=w116, y=w112) -> (x-y=w111:dbl[])
            n28 = Multiply(x=w110, y=2.0) -> (x*y=w105:dbl)
            n29 = Absolute Value(x=w111) -> (abs(x)=w108:dbl[])
            n30 = Multiply(x=w105, y=w108) -> (x*y=w104:dbl[])
            n31 = Subtract(x=w106, y=w104) -> (x-y=w103:dbl[])
          }
        }
        n32 = Equal To 0?(x=w63) -> (x = 0?=w66:bool)
        n33 = Select(t=TRUE, s=w66, f=FALSE) -> (s? t:f=w55:bool)
        n34 = Index Array(array=w59) -> (element #1=w51:dbl, element #2=w50:dbl)  [unwired: 2 in]
        n35 = Multiply(x="Single Frequency (MHz)", y=1000000.0) -> (x*y=w38:dbl)
        n36 = case shown="\"Channel CH0 constant\"" "Channel - Constant" {
          tunnel: w38 -> [w80 w81]
          tunnel: [w80 w83] -> w57
          tunnel: [w80 w84] -> w56
          tunnel: w55 -> [w79 w82]
          tunnel: [w79 w85] -> w54
          tunnel: TRUE -> [w78 w85]
          tunnel: [w78 w82] -> w52
          tunnel: w51 -> [w77 w84]
          tunnel: w50 -> [w76 w83]
          tunnel: [w77 w81] -> w49
          tunnel: [w76 w81] -> w48
          frame "Channel CH1 constant", Default {
          }
          frame "Channel CH0 constant" {
          }
        }
        n37 = Bundle(0, w43, "time tolerance"=w73, w52, "Amplitude (Ch 0)"="Amplitude (Ch 0)", "Phase (Ch 0)"="Phase (Ch 0)", w49, w48, w54, "Amplitude (Ch 1)"="Amplitude (Ch 1)", "Phase (Ch 1)"="Phase (Ch 1)", w56, w57) -> (w75:T10)  [unwired: 1 in]
        n38 = Build Array(w75) -> (w47:T11)
        n39 = Build Array (concatenate)(w46, w47) -> (w45:T12)
      }
    }
  }
  n40 = flat-sequence {
    tunnel: w20 -> [w118]
    tunnel: [w119] -> w22
    tunnel: w22 -> [w127]
    tunnel: [w127] -> w21
    tunnel: w21 -> [w131]
    tunnel: [w131] -> w12
    frame #0 {
      # "Input: read settings from xml file\nor generate data with function\nor use manual input from array"
      n41 = case shown="\"Read from file\"" "Data source" {
        tunnel: w118 -> [w122 w124 _]
        tunnel: [w121 w124 w125] -> w119
        frame "Read from file" {
          n42 = call-poly <vilib>:"Read From XML File.vi"("XML File Path"="XML File Path READ (if data source = read from file)") -> ("XML Elements"=w123:string)  [unwired: 8 in, 2 out]
          n43 = Unflatten From XML(xml string=w123, type=w122) -> (value=w121:T9)  [unwired: 1 in, 1 out]
          n44 = property on="Control Elements Array" class="Arr (strict)"("Value"=w121) -> ()  [unwired: 2 in, 2 out]
        }
        frame "Generate data with function" {
